vi "End.vi"   [LabVIEW 2018, in "Toolkit.lvlib" / "Writer.lvclass"]
doc: "Finishes encoding LabVIEW types and values to MessagePack data. This must be called after writing all of the data to free resources, allow reuse of the object, and obtain the encoded MessagePack data."
uses:
  Writer.lvclass
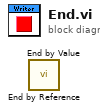
[diagram p0: block diagram]
diagram:
  n1 = call "End by Reference.vi"() -> ()  [unwired: 9 in, 3 out]
  n2 = call "End by Value.vi"() -> ()  [unwired: 9 in, 3 out]
